vi "FindTopasDevice.vi"(8 "error in (no error)":errorcluster, 10 "Serial number":string="Orpheus-HP-Demo-8047") -> (0 "error out":errorcluster, 3 "TopasDevice":refnum<k24>)   [LabVIEW 2017]
uses:
  D:/upwork/Laser Measurement Tool/Topas4PublicAPI/NET_SDK/Topas4Lib.dll
  Topas4PublicAPI/NET_SDK/Topas4Lib.dll
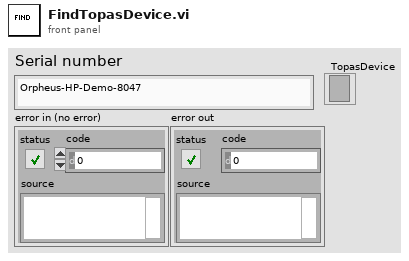
[diagram p1: front panel]
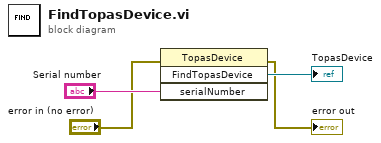
[diagram p0: block diagram]
diagram:
  n1 = invoke class="TopasDevice" method="FindTopasDevice"(error in="error in (no error)", "serialNumber"="Serial number") -> (error out=→"error out":errorcluster, "FindTopasDevice"=→"TopasDevice":refnum<k24>)  [unwired: 2 in, 2 out]
